vi "mqttCmdAcknowledge.vi"(0 "mqttConnect in":refnum<class "ConnectMqttMsg.lvclass">, 11 "error in (no error)":errorcluster) -> (4 "mqttConnect out":refnum<class "ConnectMqttMsg.lvclass">, 8 "notification":T1, 15 "error out":errorcluster)   [LabVIEW 2020, in "ConnectMqttMsg.lvclass"]
uses:
  ConnectMqttMsg.lvclass
  mqttTypedef/mqttRXdataCluster.ctl
  mqttTypedef/mqttFixedHeaderResponse.ctl
  mqttTypedef/mqttQOSlevel.ctl
  mqttTypedef/mqttMessageType.ctl
  mqttTypedef/mqttConnectionStatus.ctl
  ConnectMqttMsg.lvclass/ConnectMqttMsg.ctl
  mqtt.lvclass
panel:
  out "Success":bool
  out "payload (HEX)":u8[](array[numeric]) format="%02x"
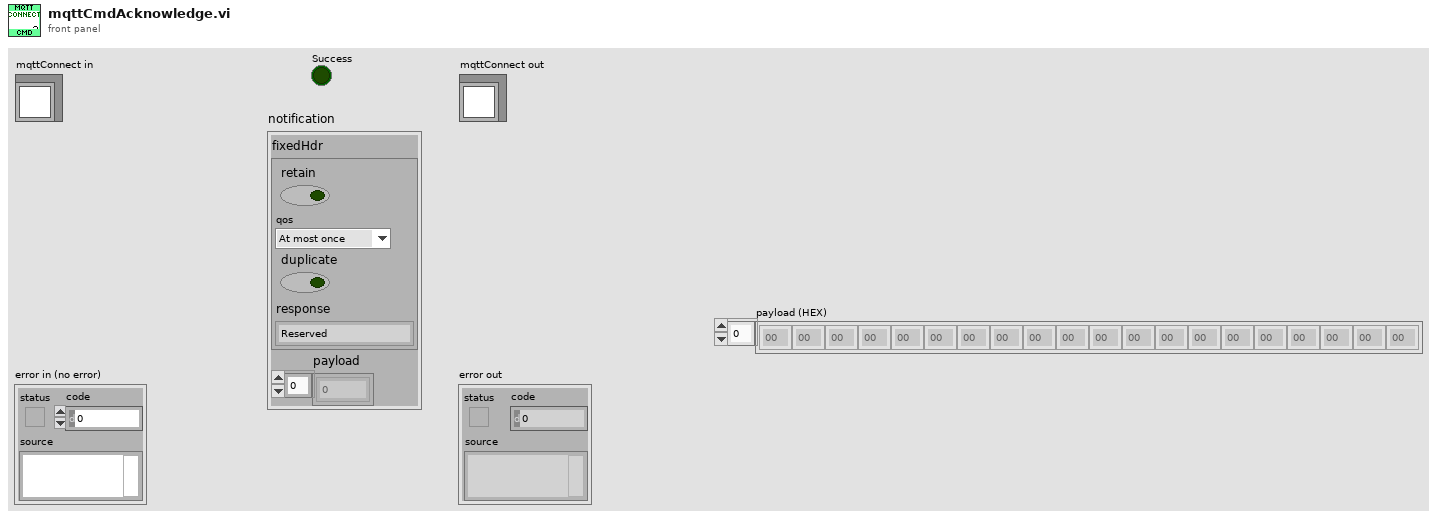
[diagram p1: front panel]
types:
  T1 = typedef "mqtt.lvclass/mqttRXdataCluster.ctl" = cluster{"fixedHdr":T2, "payload":u8[]}
  T2 = typedef "mqtt.lvclass/mqttFixedHeaderResponse.ctl" = cluster{"retain":bool, "qos":T3, "duplicate":bool, "response":T4}
  T3 = typedef "mqtt.lvclass/mqttQOSlevel.ctl" = enum8{"At most once", "At least once", "Exactly once", "Reserved"}
  T4 = typedef "mqtt.lvclass/mqttMessageType.ctl" = enum32{"Reserved", "CONNECT", "CONNACK", "PUBLISH", "PUBACK", "PUBREC", "PUBREL", "PUBCOMP", "SUBSCRIBE", "SUBACK", "UNSUBSCRIBE", "UNSUBACK", "PINGREQ", "PINGRESP", "DISCONNECT", "Reserved2"}
  T5 = typedef "mqtt.lvclass/mqttConnectionStatus.ctl" = enum16{"Connection accepted", "Connection refused: unacceptable protocol version", "Connection refused: identifier rejected", "Connection refused: Server unavailable", "Connection refused: bad user name or password", "Connection refused: not authorized"}
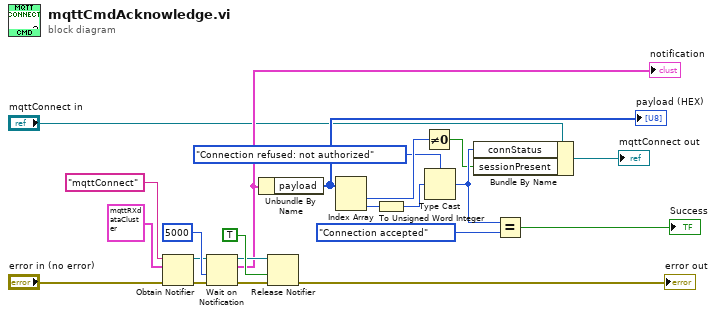
[diagram p0: block diagram]
diagram:
  n1 = Obtain Notifier(name (unnamed)="mqttConnect", notification data type=T1 {"fixedHdr"={"retain"=FALSE, "qos"=enum."At most once", "duplicate"=FALSE, "response"=enum."Reserved"}, "payload"=[]} ("output cluster"), error in (no error)="error in (no error)") -> (notifier out=w18:refnum<notifier>, error out=w17:errorcluster)  [unwired: 1 in, 1 out]
  n2 = Wait on Notification(notifier=w18, timeout in ms (-1)=5000, error in (no error)=w17) -> (notifier out=w21:refnum<notifier>, notification=w9:T1, error out=w20:errorcluster)  [unwired: 1 in, 1 out]
  "notification" <- w9
  n3 = Unbundle By Name(w9) -> ("payload"=w8:u8[])
  "payload (HEX)" <- w8
  n4 = Release Notifier(notifier=w21, force destroy? (F)=TRUE, error in (no error)=w20) -> (error out=→"error out":errorcluster)  [unwired: 2 out]
  n5 = Index Array(array=w8) -> (element #1=w13:u8, element #2=w11:u8)  [unwired: 2 in]
  n6 = To Unsigned Word Integer(number=w11) -> (unsigned 16bit integer=w10:u16)
  n7 = Not Equal To 0?(x=w13) -> (x != 0?=w1:bool)
  n8 = Type Cast(type=mqttConnectionStatus."Connection refused: not authorized" ("connStatus"), x=w10) -> (*(type *) &x=w2:T5)
  n9 = Bundle By Name(cluster="mqttConnect in", "connStatus"=w2, "sessionPresent"=w1) -> (→"mqttConnect out":refnum<class "ConnectMqttMsg.lvclass">)
  n10 = Equal?(x=w2, y=mqttConnectionStatus."Connection accepted") -> (x = y?=→"Success":bool)
